vi "Polygon Points to XY arrays.vi"(11 "Polygon Points":T1[](array[typedef]) {"Latitude" format="%#_10g"; "Longitude" format="%#_10g"}) -> (2 "Y Array":dbl[](array[numeric]), 3 "X Array":dbl[](array[numeric]))   [LabVIEW 2014]
uses:
  Lat Long Conversion/Controls/PointLatLon.ctl
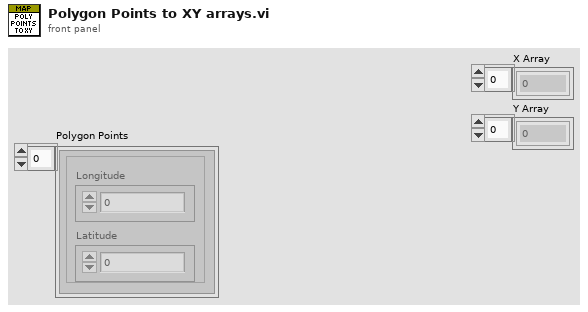
[diagram p1: front panel]
types:
  T1 = typedef "PointLatLon.ctl" = cluster{"Longitude":dbl, "Latitude":dbl}
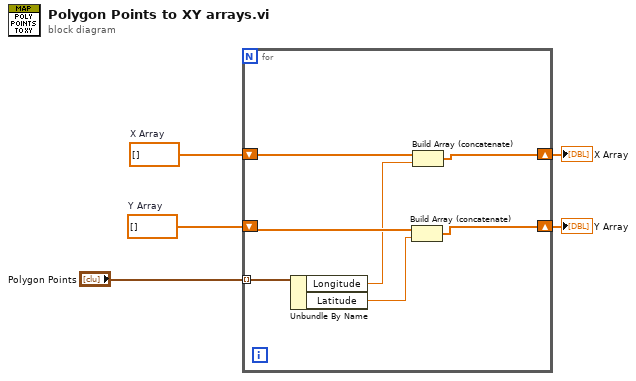
[diagram p0: block diagram]
diagram:
  w3 = dbl[] []  # Y Array
  w4 = dbl[] []  # X Array
  n1 = for {
    tunnel: "Polygon Points" -> [w12] mode=indexing
    shift-right: [w6] -> w2
    shift-left: w4 -> [w11]
    shift-right: [w7] -> w1
    shift-left: w3 -> [w10]
    n2 = Unbundle By Name(w12) -> ("Longitude"=w9:dbl, "Latitude"=w8:dbl)
    n3 = Build Array (concatenate)(w10, w8) -> (w7:dbl[])
    n4 = Build Array (concatenate)(w11, w9) -> (w6:dbl[])
  }
  "X Array" <- w2
  "Y Array" <- w1
